vi "An_sync_block_sort_New.vi"(6 "BSA 2":dbl[][](array[numeric]) format="%.3f", 9 "BSA 1":dbl[][](array[numeric]) format="%.3f") -> (0 "Analogue Sync Index":i32[](array[numeric]), 1 "BSA 2 Sync":dbl[][](array[numeric]) format="%.3f", 3 "BSA 1 Sync":dbl[][](array[numeric]) format="%.3f", 4 "No of good samples":i32=1, 5 "No of slips":i32=1)   [LabVIEW 2020]
uses:
  Globals/LDA_global.vi
panel:
  out "Output":dbl[](graph)
  out "Input":dbl[](graph)
  out "Slipped":bool
  out "TIME MARGIN":dbl format="%.2f"
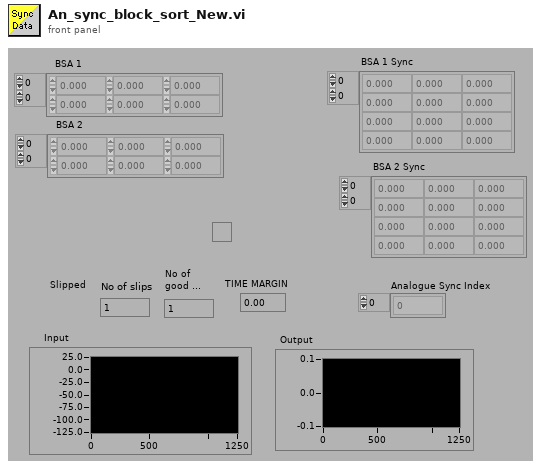
[diagram p1: front panel]
types:
  T1 = typedef "LDA_Channel.ctl" = cluster{"Wavelength (nm)":dbl, "Vel Comp":string, "Max Velocity":dbl, "Min Velocity":dbl, "Max Record length":u16, "Signal gain (dB)":i16, "High voltage":i16, "Optics Conversion Factor":dbl, "Min Record length":u16, "Multiply Velocity by -1":bool, "Signal to Noise Ratio":string, "Validation Ratio":string, "Probe":string, "Laser":string, "BSA":string, "Lense":string, "Beam Separation (mm)":dbl, "Focal Length (mm)":dbl, "COLOUR":u32, "BSA IP":string, "Velocity Range (m/s)":dbl, "Centre Velocity (m/s)":dbl, "Unshifted mW":dbl, "Shifted mW":dbl, "Bandwidth Hz":dbl, "Req Sampling Rate Hz":dbl, "Ch":i32, "CenterFreq Hz":dbl, "Laser IP":string}
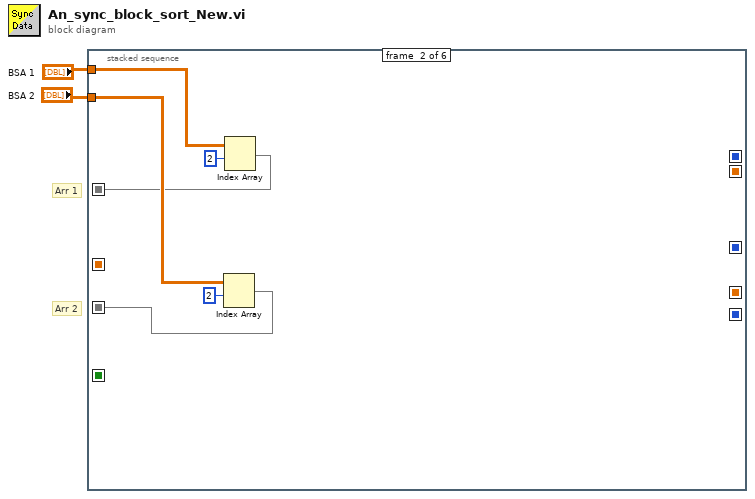
[diagram p0: block diagram]
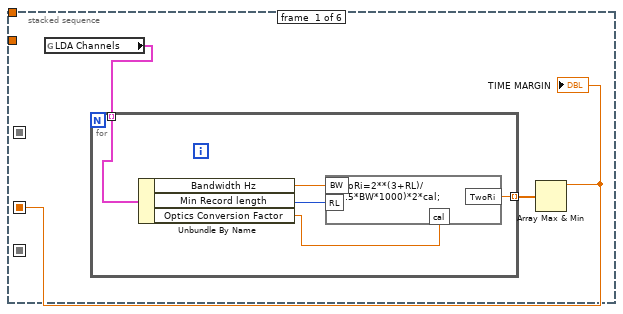
[diagram p2: hidden frame]
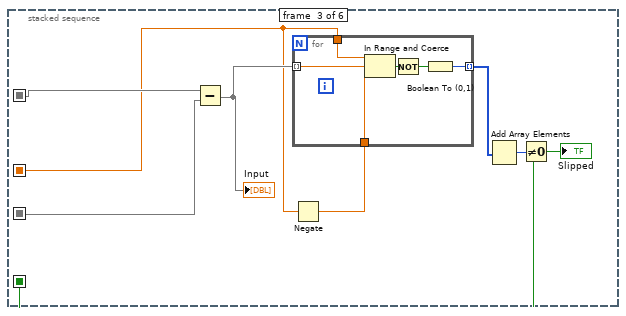
[diagram p3: hidden frame]
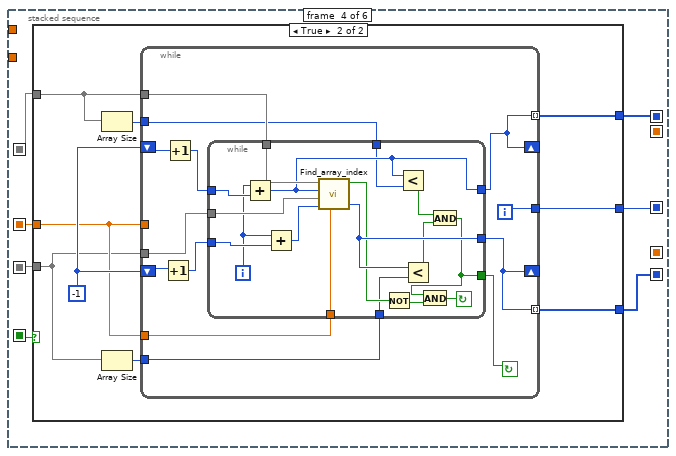
[diagram p4: hidden frame]
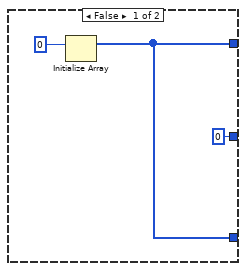
[diagram p5: hidden frame]
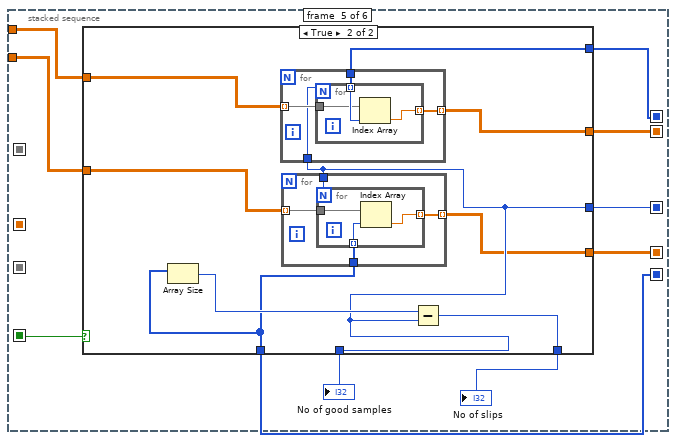
[diagram p6: hidden frame]
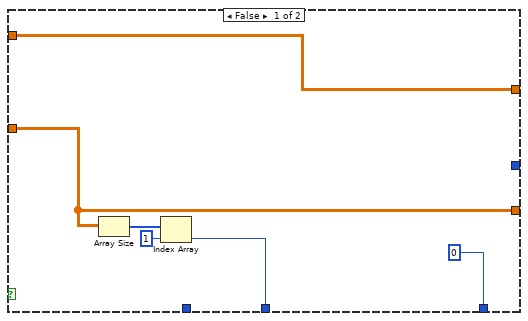
[diagram p7: hidden frame]
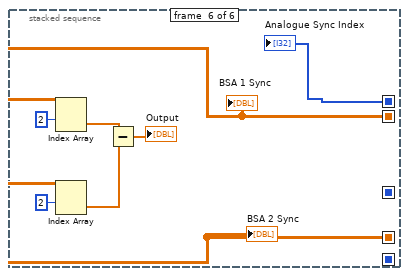
[diagram p8: hidden frame]
diagram:
  # "Arr 1"
  # "Arr 2"
  n1 = stacked-sequence {
    seq-local: [_ _ _ w37 _ _] -> [_ _ _ _ w88 w119]
    seq-local: [_ _ _ w36 _ _] -> [_ _ _ _ w89 _]
    seq-local: [_ _ w22 _ _ _] -> [_ _ _ w35 w80 _]
    seq-local: [_ _ _ _ w82 _] -> [_ _ _ _ _ w123]
    seq-local: [_ w12 _ _ _ _] -> [_ _ w18 w34 _ _]
    seq-local: [_ w11 _ _ _ _] -> [_ _ w19 w33 _ _]
    seq-local: [_ _ _ w31 _ _] -> [_ _ _ _ w85 _]
    seq-local: [_ _ _ _ w81 _] -> [_ _ _ _ _ w120]
    seq-local: [w4 _ _ _ _ _] -> [_ _ w17 w32 _ _]
    tunnel: "BSA 1" -> [_ w16 _ _ w84 _]
    tunnel: "BSA 2" -> [_ w13 _ _ w83 _]
    frame #0 {
      n2 = global read "LDA_global.vi" "LDA Channels"() -> (w3:T1[])
      n3 = for {
        tunnel: [w10] -> w5 mode=indexing
        tunnel: w3 -> [w9] mode=indexing
        n4 = Unbundle By Name(w9) -> ("Bandwidth Hz"=w8:dbl, "Min Record length"=w7:u16, "Optics Conversion Factor"=w6:dbl)
        n5 = formula code="TwoRi=2**(3+RL)/(1.5*BW*1000)*2*cal;"("BW"=w8, "RL"=w7, "cal"=w6) -> ("TwoRi"=w10:dbl)
      }
      n6 = Array Max & Min(array=w5) -> (max value=w4:dbl)  [unwired: 3 out]
      "TIME MARGIN" <- w4
    }
    frame #1 {
      n7 = Index Array(array=w13, index (row)=2 ("Index")) -> (element=w11:dbl[])  [unwired: 1 in]
      n8 = Index Array(array=w16, index (row)=2 ("Index")) -> (element=w12:dbl[])  [unwired: 1 in]
    }
    frame #2 {
      n9 = Subtract(x=w18, y=w19) -> (x-y=w20:dbl[])
      "Input" <- w20
      n10 = Negate(x=w17) -> (-x=w24:dbl)
      n11 = for {
        tunnel: w17 -> [w30]
        tunnel: w24 -> [w29]
        tunnel: w20 -> [w28] mode=indexing
        tunnel: [w26] -> w21 mode=indexing
        n12 = In Range and Coerce(upper limit=w30, x=w28, lower limit=w29) -> (In Range?=w25:bool)  [unwired: 1 out]
        n13 = Not(x=w25) -> (.not. x?=w27:bool)
        n14 = Boolean To (0,1)(Boolean=w27) -> (0, 1=w26:i16)
      }
      n15 = Add Array Elements(numeric array=w21) -> (sum=w23:i16)
      n16 = Not Equal To 0?(x=w23) -> (x != 0?=w22:bool)
      "Slipped" <- w22
    }
    frame #3 {
      n17 = case shown="True" w35 {
        tunnel: w33 -> [_ w42]
        tunnel: w34 -> [_ w45]
        tunnel: [w39 w48] -> w37
        tunnel: [w39 w47] -> w36
        tunnel: w32 -> [_ w43]
        tunnel: [0 w46] -> w31
        frame False {
          n18 = Initialize Array(0) -> (w39:i32[])  [unwired: 1 out]
        }
        frame True {
          w49 = -1
          n19 = Array Size(array=w45) -> (size(s)=w44:i32)
          n20 = Array Size(array=w42) -> (size(s)=w41:i32)
          n21 = while {
            tunnel: w41 -> [w50]
            tunnel: w43 -> [w58]
            tunnel: w44 -> [w52]
            tunnel: [w60] -> w46
            tunnel: w43 -> [_]
            tunnel: [w56] -> w48 mode=indexing
            tunnel: [w53] -> w47 mode=indexing
            shift-left: w49 -> [w62]
            shift-right: [w53] -> _
            shift-left: w49 -> [w61]
            shift-right: [w56] -> _
            tunnel: w42 -> [w55]
            tunnel: w45 -> [w59]
            i -> [w60]
            stop <- w51 continue-if-true
            n22 = Increment(x=w62) -> (x+1=w54:i32)
            n23 = Increment(x=w61) -> (x+1=w57:i32)
            n24 = while {
              tunnel: w50 -> [w63]
              tunnel: [w65] -> w51
              tunnel: w52 -> [w64]
              tunnel: w59 -> [w73]
              tunnel: w58 -> [w74]
              tunnel: [w71] -> w53
              tunnel: [w72] -> w56
              tunnel: w55 -> [w77]
              tunnel: w54 -> [w78]
              tunnel: w57 -> [w79]
              i -> [w76]
              stop <- w66 continue-if-true
              n25 = Add(x=w76, y=w79) -> (x+y=w72:i32)
              n26 = Add(x=w76, y=w78) -> (x+y=w75:i32)
              n27 = call "Find_array_index.vi"("TIME MARGIN"=w74, "AT 2 index"=w75, "AT 2 array"=w77, "AT 1 index"=w72, "AT 1 array"=w73) -> ("AT 2 index out"=w71:i32, "Found matching Element in array 2"=w68:bool)  [unwired: 4 out]
              n28 = Not(x=w68) -> (.not. x?=w67:bool)
              n29 = Less?(x=w72, y=w64) -> (x < y?=w69:bool)
              n30 = Less?(x=w71, y=w63) -> (x < y?=w70:bool)
              n31 = And(x=w69, y=w70) -> (x .and. y?=w65:bool)
              n32 = And(x=w65, y=w67) -> (x .and. y?=w66:bool)
            }
          }
        }
      }
    }
    frame #4 {
      n33 = case shown="True" w80 {
        tunnel: w88 -> [_ w104]
        tunnel: w89 -> [_ w98]
        tunnel: [w90 w101] -> w87
        tunnel: [0 w102] -> w86
        tunnel: w85 -> [_ w101]
        tunnel: w84 -> [w94 w100]
        tunnel: w83 -> [w91 w99]
        tunnel: [w94 w97] -> w82
        tunnel: [w91 w96] -> w81
        frame False {
          n34 = Array Size(array=w91) -> (size(s)=w93:i32[])
          n35 = Index Array(array=w93, index=1 ("Index")) -> (element=w90:i32)
        }
        frame True {
          n36 = Array Size(array=w98) -> (size(s)=w103:i32)
          n37 = for {
            tunnel: w104 -> [w115]
            tunnel: w100 -> [w114] mode=indexing
            tunnel: [w113] -> w97 mode=indexing
            tunnel: w101 -> [w112]
            n38 = for {
              N: w112 -> [_]
              tunnel: w115 -> [w118] mode=indexing
              tunnel: w114 -> [w117]
              tunnel: [w116] -> w113 mode=indexing
              n39 = Index Array(array=w117, index=w118) -> (element=w116:dbl)
            }
          }
          n40 = for {
            tunnel: w99 -> [w108] mode=indexing
            tunnel: w98 -> [w107]
            tunnel: [w106] -> w96 mode=indexing
            tunnel: w101 -> [w105]
            n41 = for {
              N: w105 -> [_]
              tunnel: w108 -> [w111]
              tunnel: w107 -> [w110] mode=indexing
              tunnel: [w109] -> w106 mode=indexing
              n42 = Index Array(array=w111, index=w110) -> (element=w109:dbl)
            }
          }
          n43 = Subtract(x=w103, y=w101) -> (x-y=w102:i32)
        }
      }
      "No of slips" <- w86
      "No of good samples" <- w87
    }
    frame #5 {
      n44 = Index Array(array=w123, index (row)=2 ("Index")) -> (element=w126:dbl[])  [unwired: 1 in]
      n45 = Index Array(array=w120, index (row)=2 ("Index")) -> (element=w124:dbl[])  [unwired: 1 in]
      n46 = Subtract(x=w126, y=w124) -> (x-y=→"Output":dbl[])
      "BSA 1 Sync" <- w123
      "BSA 2 Sync" <- w120
      "Analogue Sync Index" <- w119
    }
  }
